vi "set magnet.vi"(8 "error in (no error)":errorcluster, 9 "Magnet field(Oe)":dbl, 11 "VISA Resource Name":refnum<visa-resource-name>) -> (0 "error out":errorcluster, 3 "dup VISA session":refnum<visa-resource-name>)   [LabVIEW 2019, in "9T cmag.lvlib"]
uses:
  9T cmag.lvlib
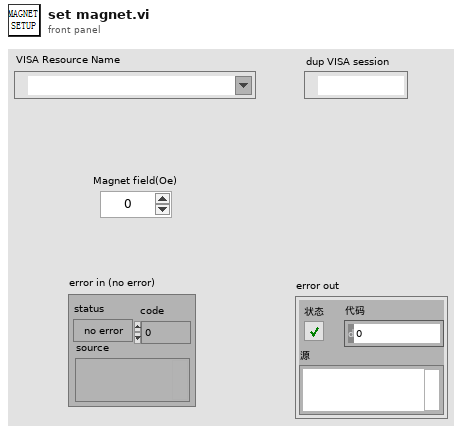
[diagram p1: front panel]
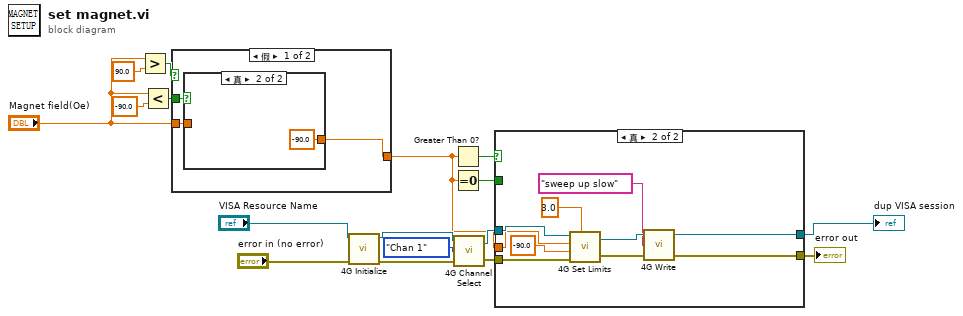
[diagram p0: block diagram]
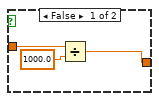
[diagram p2: hidden frame]
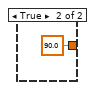
[diagram p3: hidden frame]
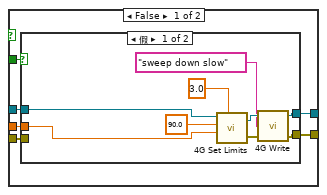
[diagram p4: hidden frame]
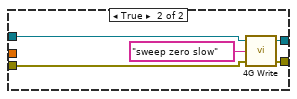
[diagram p5: hidden frame]
diagram:
  n1 = Greater?(x="Magnet field(Oe)", y=90.0) -> (0:w5:bool)
  n2 = Less?(x="Magnet field(Oe)", y=-90.0) -> (x < y?=w1:bool)
  n3 = case shown="假" w5 {
    tunnel: "Magnet field(Oe)" -> [w20 _]
    tunnel: [w19 90.0] -> w4
    tunnel: w1 -> [w18 _]
    frame False {
      n4 = case shown="真" w18 {
        tunnel: w20 -> [w22 _]
        tunnel: [w21 -90.0] -> w19
        frame False {
          n5 = Divide(x=w22, y=1000.0) -> (x/y=w21:dbl)
        }
        frame True {
        }
      }
    }
    frame True {
    }
  }
  n6 = call "4G Initialize.vi"("error in (no error)"="error in (no error)", "VISA Resource Name"="VISA Resource Name") -> ("error out"=w7:errorcluster, "VISA Resource Out"=w8:refnum<visa-resource-name>)  [unwired: 4 in]
  n7 = Greater Than 0?(x=w4) -> (x > 0?=w12:bool)
  n8 = Equal To 0?(x=w4) -> (x = 0?=w11:bool)
  n9 = call "4G Channel Select.vi"("error in (no error)"=w7, "Channel"=enum16{"Chan 1", "Chan 2"}."Chan 1", "VISA session"=w8) -> ("error out"=w15:errorcluster, "VISA session out"=w16:refnum<visa-resource-name>)
  n10 = case shown="真" w12 {
    tunnel: w16 -> [w31 w55]
    tunnel: w4 -> [w30 w53]
    tunnel: [w29 w49] -> w14
    tunnel: w15 -> [w26 w51]
    tunnel: [w28 w47] -> w13
    tunnel: w11 -> [w27 _]
    frame False {
      n11 = case shown="假" w27 {
        tunnel: w31 -> [w40 w45]
        tunnel: w30 -> [w39 _]
        tunnel: [w34 w44] -> w29
        tunnel: [w33 w43] -> w28
        tunnel: w26 -> [_ w42]
        frame False {
          n12 = call "4G Set Limits.vi"("VISA session"=w40, "upper limit"=90.0, "lower limit"=w39, "voltage limit"=3.0) -> ("dup VISA session"=w36:refnum<visa-resource-name>, "error out"=w35:errorcluster)  [unwired: 1 in]
          n13 = call "4G Write.vi"("error in (no error)"=w35, "write buffer (\"\")"="sweep down slow" ("write buffer (\"\")"), "VISA session"=w36) -> ("error out"=w33:errorcluster, "dup VISA session"=w34:refnum<visa-resource-name>)  [unwired: 1 out]
        }
        frame True {
          n14 = call "4G Write.vi"("error in (no error)"=w42, "write buffer (\"\")"="sweep zero slow" ("write buffer (\"\")"), "VISA session"=w45) -> ("error out"=w43:errorcluster, "dup VISA session"=w44:refnum<visa-resource-name>)  [unwired: 1 out]
        }
      }
    }
    frame True {
      n15 = call "4G Set Limits.vi"("VISA session"=w55, "upper limit"=w53, "lower limit"=-90.0, "error in (no error)"=w51, "voltage limit"=3.0) -> ("dup VISA session"=w50:refnum<visa-resource-name>, "error out"=w48:errorcluster)
      n16 = call "4G Write.vi"("error in (no error)"=w48, "write buffer (\"\")"="sweep up slow" ("write buffer (\"\")"), "VISA session"=w50) -> ("error out"=w47:errorcluster, "dup VISA session"=w49:refnum<visa-resource-name>)  [unwired: 1 out]
    }
  }
  "dup VISA session" <- w14
  "error out" <- w13
